vi "SID reverb.vi"(5 "sampling info":cluster{"Fs":dbl, "#s":i32}={"Fs"=44100.0, "#s"=50}, 6 "reset":bool, 9 "delay":dbl=0.995, 11 "wave in":dbl[](array[numeric])) -> (3 "wave out":dbl[](array[numeric]))   [LabVIEW 2018]
panel:
  in  "wet":dbl=0.4 format="%#_13g"
  in  "feedback":dbl=0.30000000000000004 format="%#_13g"
  in  "lp coeff":dbl=0.24999999999999997 format="%#_13g"
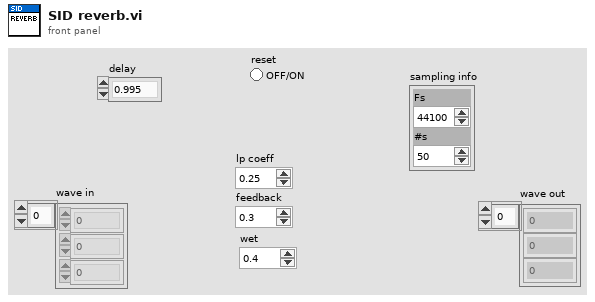
[diagram p1: front panel]
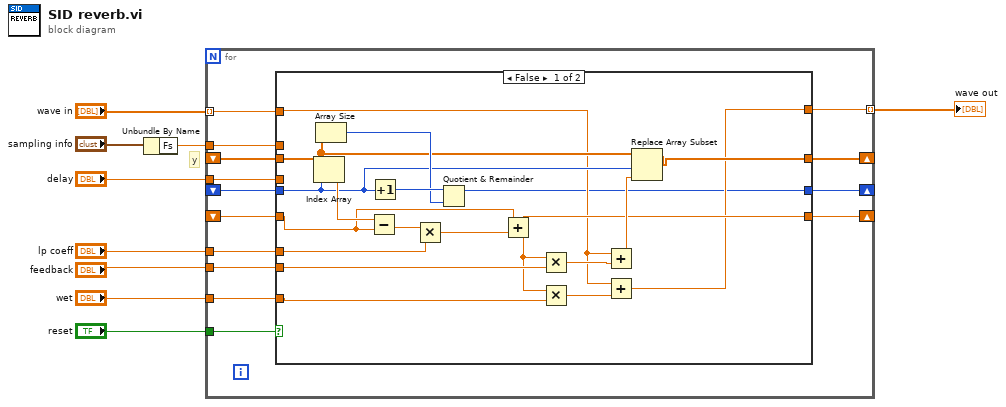
[diagram p0: block diagram]
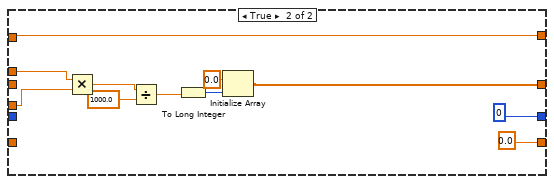
[diagram p2: hidden frame]
diagram:
  # "y"
  n1 = Unbundle By Name("sampling info") -> ("Fs"=w1:dbl)
  n2 = for {
    shift-right: [w19] -> _
    shift-left: _ -> [w22]
    shift-right: [w18] -> _
    shift-left: _ -> [w17]
    shift-right: [w13] -> _
    shift-left: _ -> [w15]
    tunnel: "wave in" -> [w16] mode=indexing
    tunnel: "lp coeff" -> [w14]
    tunnel: "reset" -> [w23]
    tunnel: "delay" -> [w21]
    tunnel: w1 -> [w20]
    tunnel: "feedback" -> [w12]
    tunnel: "wet" -> [w11]
    tunnel: [w10] -> w3 mode=indexing
    n3 = case shown="False" w23 {
      tunnel: w22 -> [w35 _]
      tunnel: w21 -> [_ w49]
      tunnel: w20 -> [_ w48]
      tunnel: [w34 w46] -> w19
      tunnel: [w24 0] -> w18
      tunnel: w17 -> [w30 _]
      tunnel: w16 -> [w26 w43]
      tunnel: w15 -> [w37 _]
      tunnel: w14 -> [w38 _]
      tunnel: [w29 0.0] -> w13
      tunnel: w12 -> [w33 _]
      tunnel: w11 -> [w28 _]
      tunnel: [w25 w43] -> w10
      frame False {
        n4 = Index Array(array=w35, index=w30) -> (element=w40:dbl)
        n5 = Array Size(array=w35) -> (size(s)=w41:i32)
        n6 = Subtract(x=w40, y=w37) -> (x-y=w39:dbl)
        n7 = Increment(x=w30) -> (x+1=w42:i32)
        n8 = Multiply(x=w39, y=w38) -> (x*y=w36:dbl)
        n9 = Quotient & Remainder(x=w42, y=w41) -> (x-y*floor(x/y)=w24:i32)  [unwired: 1 out]
        n10 = Add(x=w37, y=w36) -> (x+y=w29:dbl)
        n11 = Multiply(x=w29, y=w33) -> (x*y=w32:dbl)
        n12 = Multiply(x=w29, y=w28) -> (x*y=w27:dbl)
        n13 = Add(x=w26, y=w32) -> (x+y=w31:dbl)
        n14 = Add(x=w26, y=w27) -> (x+y=w25:dbl)
        n15 = Replace Array Subset(array=w35, new element=w31, index=w30) -> (w34:dbl[])
      }
      frame True {
        n16 = Multiply(x=w48, y=w49) -> (x*y=w51:dbl)
        n17 = Divide(x=w51, y=1000.0) -> (x/y=w52:dbl)
        n18 = To Long Integer(number=w52) -> (32bit integer=w53:i32)
        n19 = Initialize Array(0.0 ("element"), w53) -> (w46:dbl[])
      }
    }
  }
  "wave out" <- w3
